vi "Global 2.vi"() -> ()   [LabVIEW 2014]
panel:
  in  "Numeric":dbl
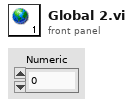
[diagram p1: front panel]
diagram:
